vi "GetDataSection.vi"(8 "error in (no error)":errorcluster caption="에러 입력(에러 없음)", 10 "SectionMap":T2, 11 "ABFFIO 입력":refnum<class "ABFFIO.lvclass">) -> (0 "error out":errorcluster caption="에러 출력", 1 "DataProperties":T1, 2 "배열":sgl[][][](array[numeric]), 3 "ABFFIO 출력":refnum<class "ABFFIO.lvclass">)   [LabVIEW 2017, in "ABFFIO.lvclass"]
uses:
  ABFFIO.lvclass
  ABFFIO.lvclass/ABFFIO.ctl
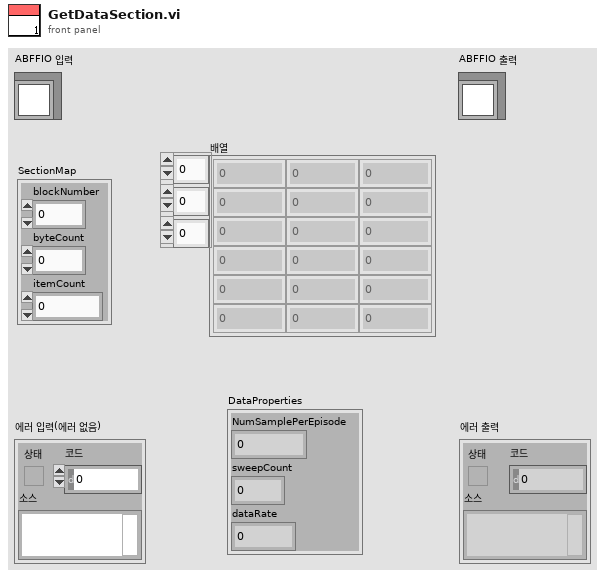
[diagram p1: front panel]
types:
  T1 = cluster{"NumSamplePerEpisode":u32, "sweepCount":u32, "dataRate":i32}
  T2 = cluster{"blockNumber":u32, "byteCount":u32, "itemCount":u32}
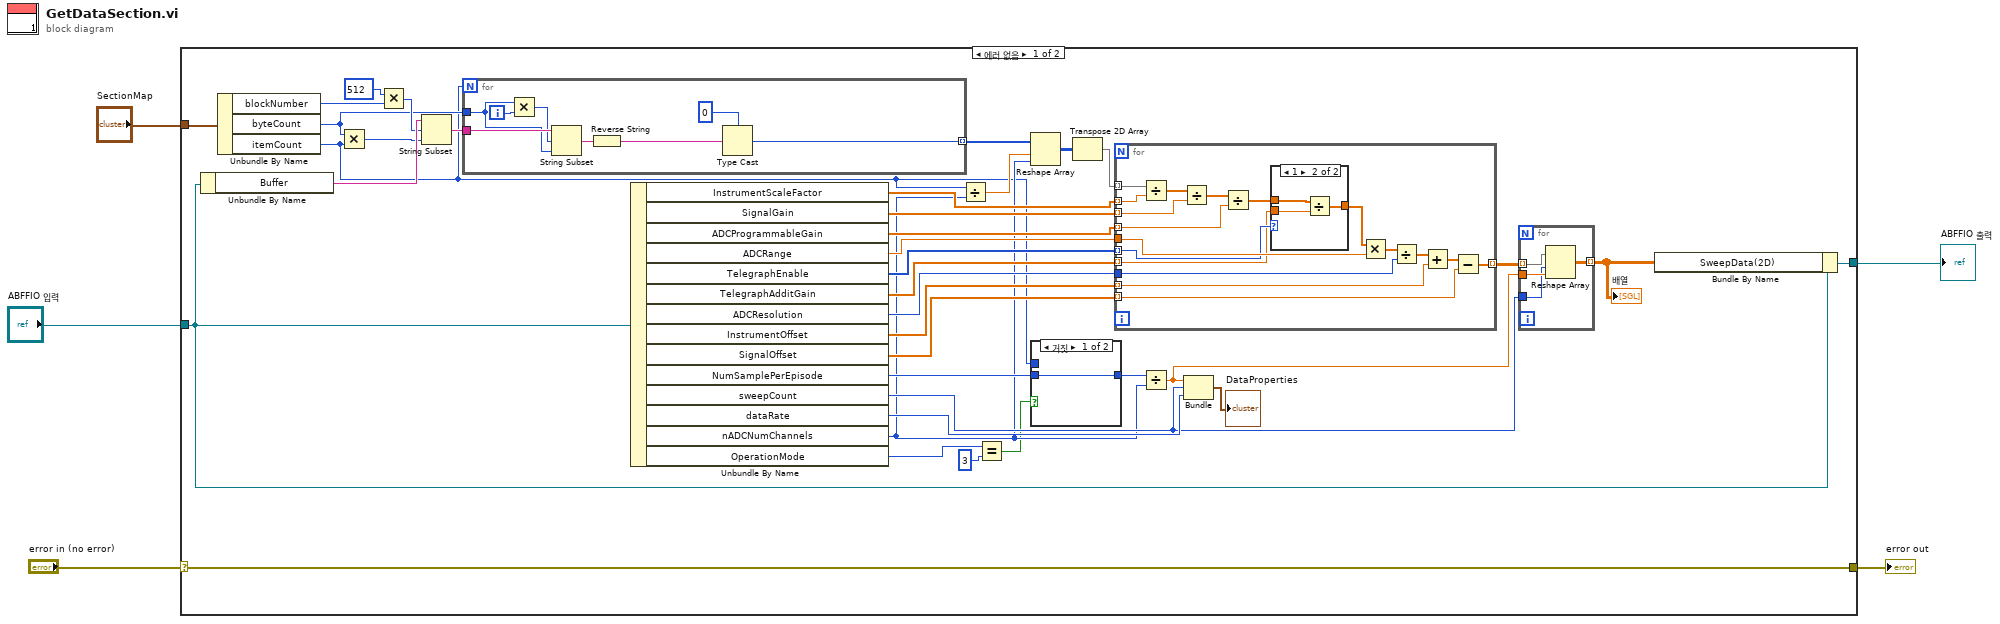
[diagram p0: block diagram]
diagram:
  n1 = case shown="에러 없음" "error in (no error)" {
    selector: "error in (no error)" -> [w42 w80]
    tunnel: [w42 w80] -> w4
    tunnel: [w26 w79] -> w2
    tunnel: "ABFFIO 입력" -> [w27 w79]
    tunnel: "SectionMap" -> [w41 _]
    frame No Error {
      n2 = Unbundle By Name(w27) -> ("Buffer"=w39:string)
      n3 = Unbundle By Name(w41) -> ("blockNumber"=w40:u32, "byteCount"=w34:u32, "itemCount"=w9:u32)
      n4 = Multiply(x=w34, y=w9) -> (x*y=w37:u32)
      n5 = Multiply(x=u32 512, y=w40) -> (x*y=w38:u32)
      n6 = String Subset(string=w39, offset (0)=w38, length (rest)=w37) -> (substring=w35:string)
      n7 = for {
        N: w9 -> [_]
        tunnel: w35 -> [w77]
        tunnel: w34 -> [w76]
        tunnel: [w74] -> w22 mode=indexing
        i -> [w78]
        n8 = Multiply(x=w76, y=w78) -> (x*y=w73:u32)
        n9 = String Subset(string=w77, offset (0)=w73, length (rest)=w76) -> (substring=w72:string)
        n10 = Reverse String(1:w72) -> (0:w71:string)
        n11 = Type Cast(type=i16 0 ("x"), x=w71) -> (*(type *) &x=w74:i16)
      }
      n12 = Unbundle By Name(w27) -> ("InstrumentScaleFactor"=w33:sgl[], "SignalGain"=w32:sgl[], "ADCProgrammableGain"=w31:sgl[], "ADCRange"=w30:sgl, "TelegraphEnable"=w14:u8[], "TelegraphAdditGain"=w15:sgl[], "ADCResolution"=w29:u32, "InstrumentOffset"=w28:sgl[], "SignalOffset"=w20:sgl[], "NumSamplePerEpisode"=w12:u32, "sweepCount"=w17:u32, "dataRate"=w19:i32, "nADCNumChannels"=w10:u32, "OperationMode"=w8:u8)
      n13 = Divide(x=w9, y=w10) -> (x/y=w24:dbl)
      n14 = Equal?(x=w8, y=u8 3) -> (x = y?=w6:bool)
      n15 = Reshape Array(w22, w24, w10) -> (w23:i16[][])
      n16 = case shown="거짓" w6 {
        tunnel: w12 -> [w43 _]
        tunnel: [w43 w44] -> w11
        tunnel: w9 -> [_ w44]
        frame False {
        }
        frame True {
        }
      }
      n17 = Transpose 2D Array(2D array=w23) -> (transposed array=w21:i16[][])
      n18 = for {
        tunnel: w33 -> [w66] mode=indexing
        tunnel: w32 -> [w64] mode=indexing
        tunnel: w31 -> [w63] mode=indexing
        tunnel: w30 -> [w61]
        tunnel: w29 -> [w59]
        tunnel: w28 -> [w57] mode=indexing
        tunnel: w21 -> [w56] mode=indexing
        tunnel: [w54] -> w18 mode=indexing
        tunnel: w20 -> [w53] mode=indexing
        tunnel: w15 -> [w49] mode=indexing
        tunnel: w14 -> [w52] mode=indexing
        n19 = Divide(x=w56, y=w66) -> (x/y=w65:sgl[])
        n20 = Divide(x=w65, y=w64) -> (x/y=w62:sgl[])
        n21 = Divide(x=w62, y=w63) -> (x/y=w51:sgl[])
        n22 = case shown="1" w52 {
          tunnel: w51 -> [w67 w70]
          tunnel: [w67 w68] -> w50
          tunnel: w49 -> [_ w69]
          frame 0, Default {
          }
          frame 1 {
            n23 = Divide(x=w70, y=w69) -> (x/y=w68:sgl[])
          }
        }
        n24 = Multiply(x=w50, y=w61) -> (x*y=w60:sgl[])
        n25 = Divide(x=w60, y=w59) -> (x/y=w58:sgl[])
        n26 = Add(x=w58, y=w57) -> (x+y=w55:sgl[])
        n27 = Subtract(x=w55, y=w53) -> (x-y=w54:sgl[])
      }
      n28 = Divide(x=w11, y=w10) -> (x/y=w16:dbl)
      n29 = Bundle(w16, "sweepCount"=w17, "dataRate"=w19) -> (→"DataProperties":cluster{dbl, "sweepCount":u32, "dataRate":i32})  [unwired: 1 in]
      n30 = for {
        tunnel: w18 -> [w48] mode=indexing
        tunnel: w17 -> [w45]
        tunnel: w16 -> [w46]
        tunnel: [w47] -> w13 mode=indexing
        n31 = Reshape Array(w48, w45, w46) -> (w47:sgl[][])
      }
      "배열" <- w13
      n32 = Bundle By Name(cluster=w27, "SweepData(2D)"=w13) -> (w26:refnum<class "ABFFIO.lvclass">)
    }
    frame Error {
    }
  }
  "error out" <- w4
  "ABFFIO 출력" <- w2
